vi "GeneratedGetOwnerUID.vi"(0 "Generic in":refnum<vi>) -> (1 "Cluster":cluster{bool, "UID":i32})   [LabVIEW 2013]
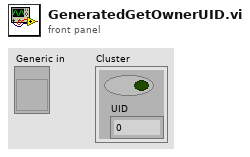
[diagram p1: front panel]
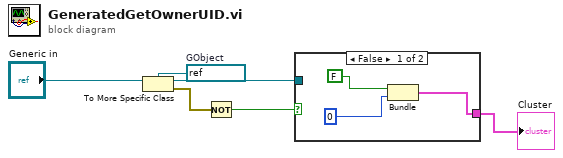
[diagram p0: block diagram]
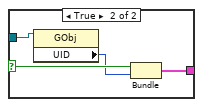
[diagram p2: hidden frame]
diagram:
  w3 = refnum<vi> refnum  # GObject
  n1 = To More Specific Class(target class=w3, reference="Generic in") -> (specific class reference=w5:refnum<vi>, error out=w1:errorcluster)  [unwired: 1 in]
  n2 = Not(x=w1) -> (.not. x?=w2:bool)
  n3 = case shown="False" w2 {
    selector: w2 -> [_ w13]
    tunnel: w5 -> [_ w12]
    tunnel: [w9 w10] -> w6
    frame False {
      n4 = Bundle(FALSE, 0) -> (w9:cluster{bool, i32})  [unwired: 1 in]
    }
    frame True {
      n5 = property class="GObj"(reference=w12) -> ("UID"=w11:i32)  [unwired: 1 in, 2 out]
      n6 = Bundle(w13, "UID"=w11) -> (w10:cluster{bool, "UID":i32})  [unwired: 1 in]
    }
  }
  "Cluster" <- w6
